vi "Clear Previous Case Data.vi"(6 "Nested Actor's Enqueuer":refnum<class "Message Enqueuer.lvclass">, 10 "error in":errorcluster) -> (2 "error out":errorcluster)   [LabVIEW 2016, in "Optimization Framework.lvlib" / "Optimization.lvclass"]
uses:
  Optimization.lvclass
  <vilib>/ActorFramework/Message Enqueuer/Message Enqueuer.lvclass
  Utilities/Delivery Notifier Handler.llb/Delivery Notifier Handler Command.ctl
  <vilib>/ActorFramework/Message Enqueuer/Message Enqueuer.lvclass/Message Enqueuer.ctl
  <vilib>/ActorFramework/Message Enqueuer/Enqueue.vi
  <vilib>/ActorFramework/Stop Msg/Stop Msg.lvclass
  C:/Program Files (x86)/National Instruments/LabVIEW 2016/vi.lib/ActorFramework/Message/Message.lvclass
  <vilib>/ActorFramework/Message Priority Queue/Priority Enqueue.vi
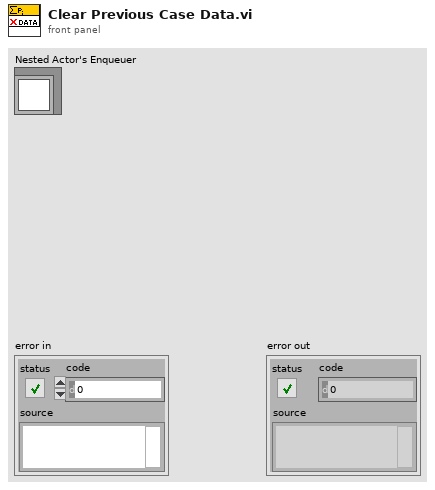
[diagram p1: front panel]
types:
  T1 = typedef "Optimization Framework.lvlib/Optimization.lvclass/Delivery Notifier Handler Command.ctl" = enum16{"Initiate", "Store", "Close All"}
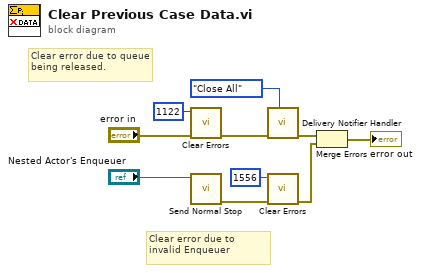
[diagram p0: block diagram]
diagram:
  # "Clear error due to invalid Enqueuer"
  # "Clear error due to queue being released."
  n1 = call <vilib>:"Clear Errors.vi"("error in (no error)"="error in", "specific error code to clear (0: all)"=1122) -> ("error out"=w5:errorcluster)  [unwired: 4 in, 1 out]
  n2 = call <vilib>:"Send Normal Stop.vi"("Message Enqueuer"="Nested Actor's Enqueuer") -> ("error out"=w10:errorcluster)  [unwired: 10 in]
  n3 = call "Delivery Notifier Handler.vi"("Command (Store)"=Delivery_Notifier_Handler_Command."Close All", "error in"=w5) -> ("error out"=w3:errorcluster)  [unwired: 9 in]
  n4 = call <vilib>:"Clear Errors.vi"("error in (no error)"=w10, "specific error code to clear (0: all)"=1556) -> ("error out"=w1:errorcluster)  [unwired: 4 in, 1 out]
  n5 = Merge Errors(w3, w1) -> (→"error out":errorcluster)
